vi "Config.vi"(8 "error in (no error)":errorcluster, 9 "Channel Name":string, 10 "Setting":T1={"Max. Volt"=10.0, "Current Limit"=0.5, "Measurement Type"=1, "Volt Level"=10.0} {"Measurement Type" items=["Voltage"=1, "Current"=0]}, 11 "Keysight 5700C in":refnum<class "Keysight 5700C.lvclass">) -> (0 "error out":errorcluster, 3 "Keysight 5700C out":refnum<class "Keysight 5700C.lvclass">)   [LabVIEW 2021, in "Concrete.lvlib" / "Keysight 5700C.lvclass"]
uses:
  Keysight 5700C.lvclass
  Keysight 5700C.lvclass/Keysight 5700C.ctl
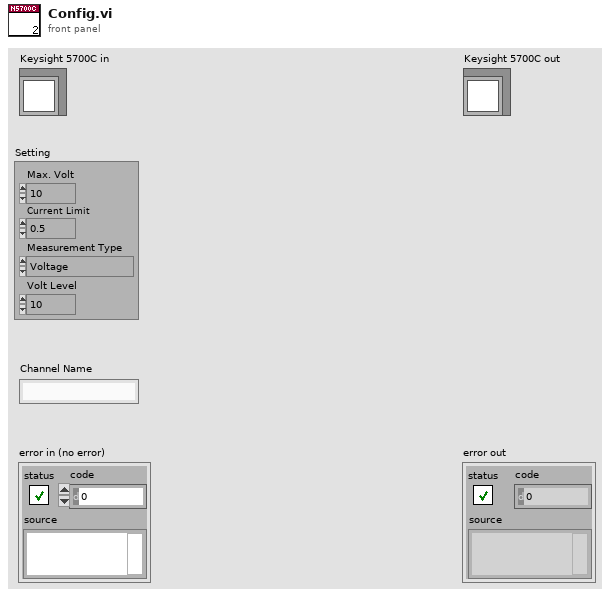
[diagram p1: front panel]
types:
  T1 = cluster{"Max. Volt":dbl, "Current Limit":dbl, "Measurement Type":i32, "Volt Level":dbl}
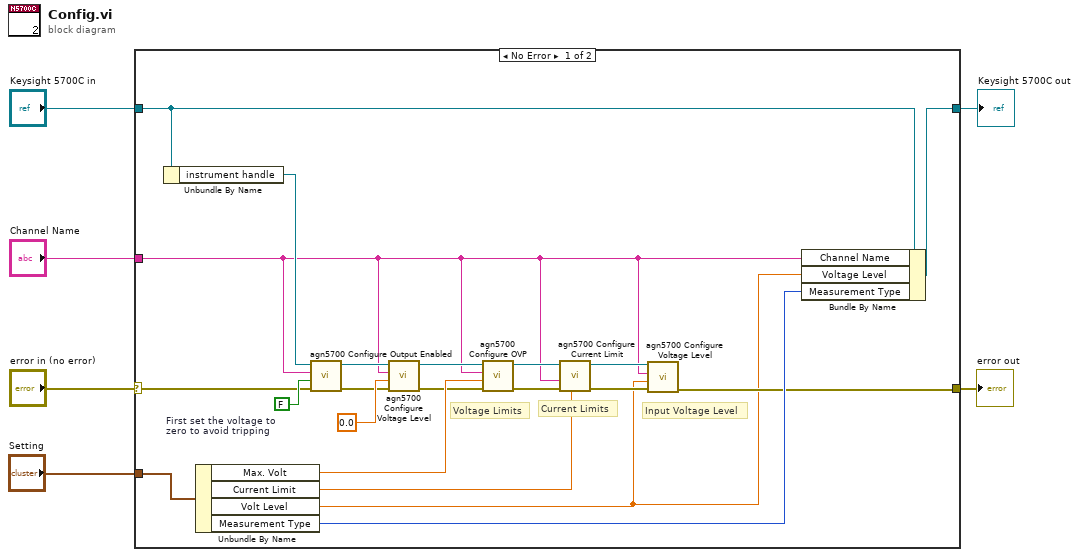
[diagram p0: block diagram]
diagram:
  n1 = case shown="No Error" "error in (no error)" {
    selector: "error in (no error)" -> [w18 w29]
    tunnel: [w8 w29] -> w5
    tunnel: [w27 w28] -> w3
    tunnel: "Keysight 5700C in" -> [w17 w28]
    tunnel: "Setting" -> [w19 _]
    tunnel: "Channel Name" -> [w9 _]
    frame No Error {
      w24 = 0.0  # First set the voltage to zero to avoid tripping
      # "Input Voltage Level"
      # "Current Limits"
      # "Voltage Limits"
      n2 = Unbundle By Name(w17) -> ("instrument handle"=w16:refnum<k15>)
      n3 = Unbundle By Name(w19) -> ("Max. Volt"=w22:dbl, "Current Limit"=w14:dbl, "Volt Level"=w7:dbl, "Measurement Type"=w15:i32)
      n4 = call <instrlib>:"agn5700 Configure Output Enabled.vi"("error in (no error)"=w18, "enabled (True)"=FALSE, "channel name (\"\")"=w9, "instrument handle"=w16) -> ("error out"=w23:errorcluster, "instrument handle out"=w25:refnum<k15>)  [unwired: 6 out]
      n5 = call <instrlib>:"agn5700 Configure Voltage Level.vi"("error in (no error)"=w23, "level (0.02)"=w24, "channel name (\"\")"=w9, "instrument handle"=w25) -> ("error out"=w13:errorcluster, "instrument handle out"=w12:refnum<k15>)  [unwired: 6 out]
      n6 = call <instrlib>:"agn5700 Configure OVP.vi"("error in (no error)"=w13, "limit (5.0)"=w22, "channel name (\"\")"=w9, "instrument handle"=w12) -> ("error out"=w20:errorcluster, "instrument handle out"=w21:refnum<k15>)  [unwired: 1 in, 5 out]
      n7 = call <instrlib>:"agn5700 Configure Current Limit.vi"("limit (0.0)"=w14, "error in (no error)"=w20, "channel name (\"\")"=w9, "instrument handle"=w21) -> ("error out"=w11:errorcluster, "instrument handle out"=w10:refnum<k15>)  [unwired: 1 in, 5 out]
      n8 = call <instrlib>:"agn5700 Configure Voltage Level.vi"("error in (no error)"=w11, "level (0.02)"=w7, "channel name (\"\")"=w9, "instrument handle"=w10) -> ("error out"=w8:errorcluster)  [unwired: 7 out]
      n9 = Bundle By Name(cluster=w17, "Channel Name"=w9, "Voltage Level"=w7, "Measurement Type"=w15) -> (w27:refnum<class "Keysight 5700C.lvclass">)
    }
    frame Error {
    }
  }
  "error out" <- w5
  "Keysight 5700C out" <- w3
